vi "Actor Core.vi"(8 "error in":errorcluster, 11 "Algorythm in":refnum<class "Algorythm.lvclass">) -> (0 "error out":errorcluster, 3 "Actor out":refnum<class "Actor.lvclass">)   [LabVIEW 2020, in "Algorythm.lvlib" / "Algorythm.lvclass"]
doc: "(<B>Filename</B>: Actor Framework.lvlib:Actor.lvclass:Actor Core.vi)\n\nReceives messages to the actor, reacts to them, and initiates any error handling that may shut the actor down.\n\nDescendant classes may override this VI to append parallel tasks for the actor to complete while it handles messages. Overrides use the Call Parent Class Method node."
uses:
  Algorythm.lvclass
  C:/Program Files (x86)/National Instruments/LabVIEW 2020/vi.lib/ActorFramework/Actor/Actor.lvclass
  <vilib>/ActorFramework/Actor/Actor.lvclass
  <vilib>/ActorFramework/Actor/Actor.lvclass/Actor.ctl
  <vilib>/ActorFramework/Message Enqueuer/Message Enqueuer.lvclass/Message Enqueuer.ctl
  Algorythm.lvclass/Algorythm.ctl
  <vilib>/Platform/TimedLoop/XDataNode/timing_clust.ctl
  <vilib>/Platform/TimedLoop/XDataNode/nitl_modes.ctl
  <vilib>/Platform/TimedLoop/XDataNode/wakeup.ctl
  Modbus/Modbus Messages/Write to Module Msg/Write to Module Msg.lvclass/Write to Module Msg.ctl
  GUI Messages/Get Alg Result Msg/Get Alg Result Msg.lvclass/Get Alg Result Msg.ctl
  <vilib>/ActorFramework/Message Enqueuer/Init from Existing Queue.vi
  <vilib>/ActorFramework/Message Enqueuer/Enqueue.vi
  Modbus/Modbus Messages/Write to Module Msg/Write to Module Msg.lvclass
  C:/Program Files (x86)/National Instruments/LabVIEW 2020/vi.lib/ActorFramework/Message/Message.lvclass
  GUI Messages/Get Alg Result Msg/Get Alg Result Msg.lvclass
  <vilib>/ActorFramework/Stop Msg/Stop Msg.lvclass
  <vilib>/Platform/TimedLoop/scheduler/LVUserAPI/_suppVIs/Create_1kHz_TSource.vi
  <vilib>/Utility/LVClass/Get LV Class Name.vi
  <resource>/AFDebug/Generate Trace for Message.vi
  <vilib>/ActorFramework/Message Priority Queue/Priority Enqueue.vi
  <vilib>/ActorFramework/Message Enqueuer/Message Enqueuer.lvclass
  <vilib>/platform/TimedLoop/XDataNode/XDataNode.xnode
  <vilib>/Platform/TimedLoop/XDataNode/XDNodeRunTimeDep.lvlib
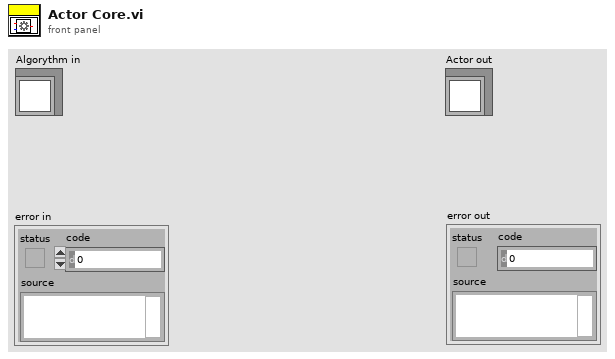
[diagram p1: front panel]
types:
  T1 = cluster{"Relay 1":bool, "Relay 2":bool, "Relay 3":bool, "Relay 4":bool, "Relay 5":bool, "Relay 6":bool, "Relay 7":bool, "Relay 8":bool}
  T2 = typedef "XDNodeRunTimeDep.lvlib/timing_clust.ctl" = cluster{"Expected End [f-1]":u64, "Actual End [f-1]":u64, "Finished Late? [f-1]":bool, "Expected End [i-1]":u64, "Actual End [i-1]":u64, "Finished Late? [i-1]":bool, "Expected Start [i]":u64, "Actual Start [i]":u64, "Expected Start [f]":u64, "Actual Start [f]":u64, "Source Name":string, "Structure Name":string, "Period":i64, "Deadline":i64, "Offset":i64, "Start":i64, "Priority":i32, "Timeout":i32, "Mode":T3, "Wakeup Reason":T4, "Error":errorcluster, "Source Type":string, "Secondary Source Type":string, "Global End Time":u64, "Global Start Time":u64, "Frame Duration":u64, "Iteration Duration":u64, "Assigned CPU":i32, "I/O Scan Engine Mode":u32}
  T3 = typedef "XDNodeRunTimeDep.lvlib/nitl_modes.ctl" = enum32{"No Change", "Process missed periods, maintain original phase", "Discard missed periods, maintain original phase", "Process missed periods, ignore original phase", "Discard missed periods, ignore original phase"}
  T4 = typedef "XDNodeRunTimeDep.lvlib/wakeup.ctl" = enum32{"Normal", "Aborted", "Asynchronous wakeup", "Timing source error", "Timed loop error", "Timeout"}
  T5 = cluster{"LDO":i32, "LAI":i32, "Control":i32, "Connect":i32}
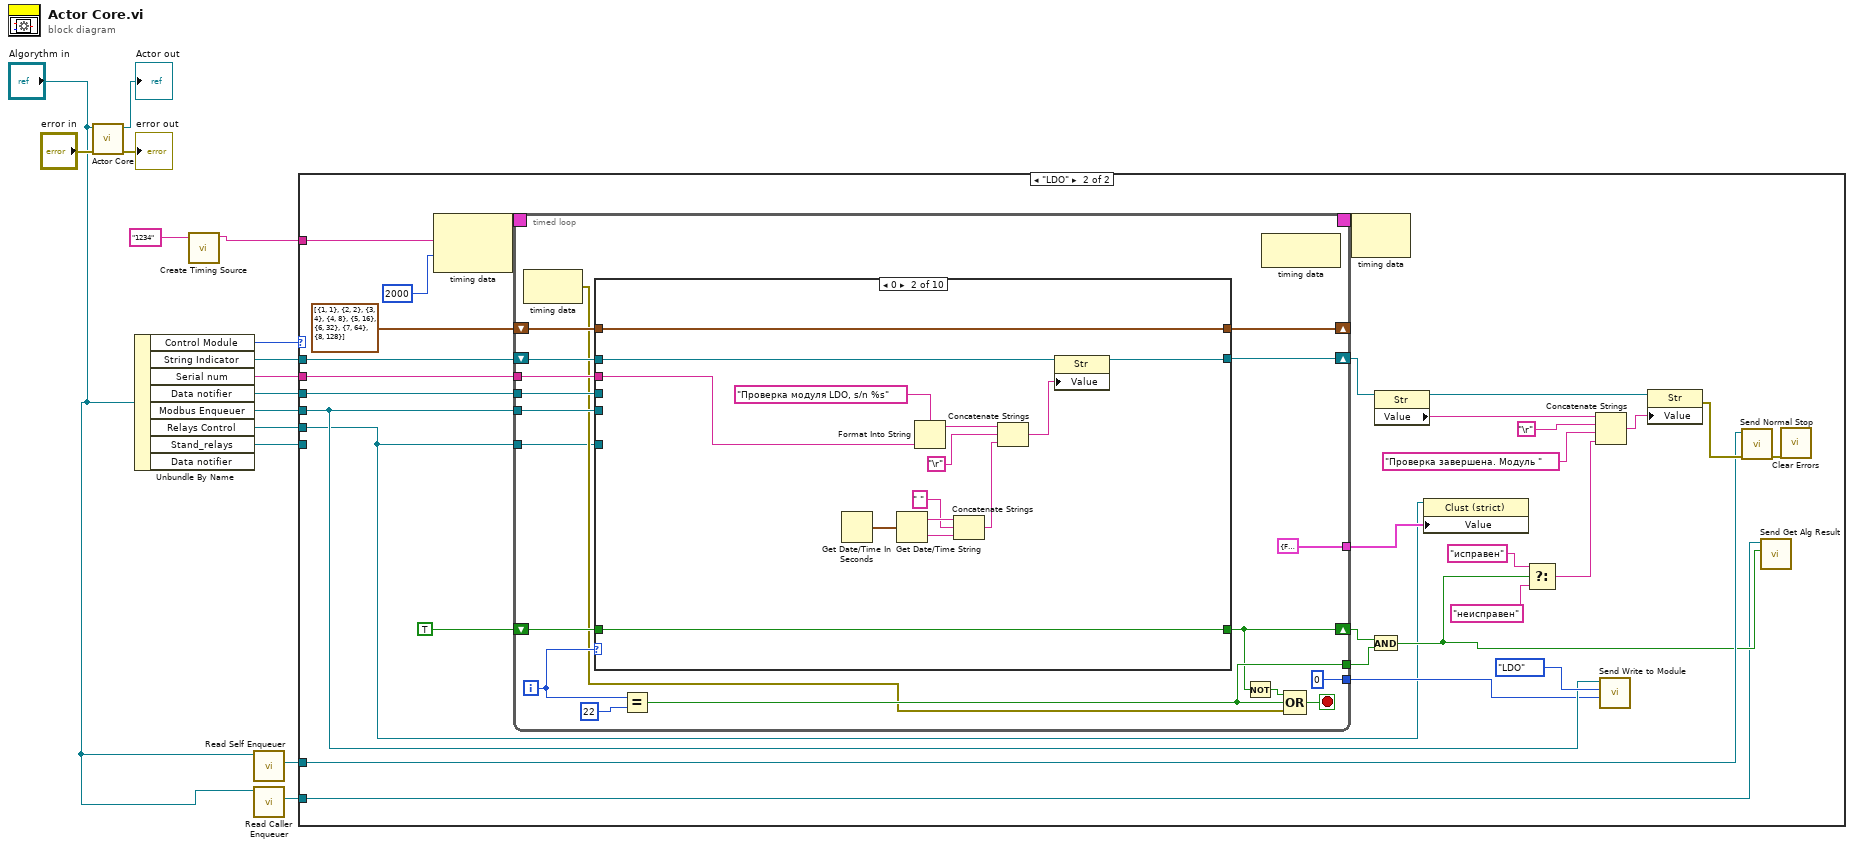
[diagram p0: block diagram]
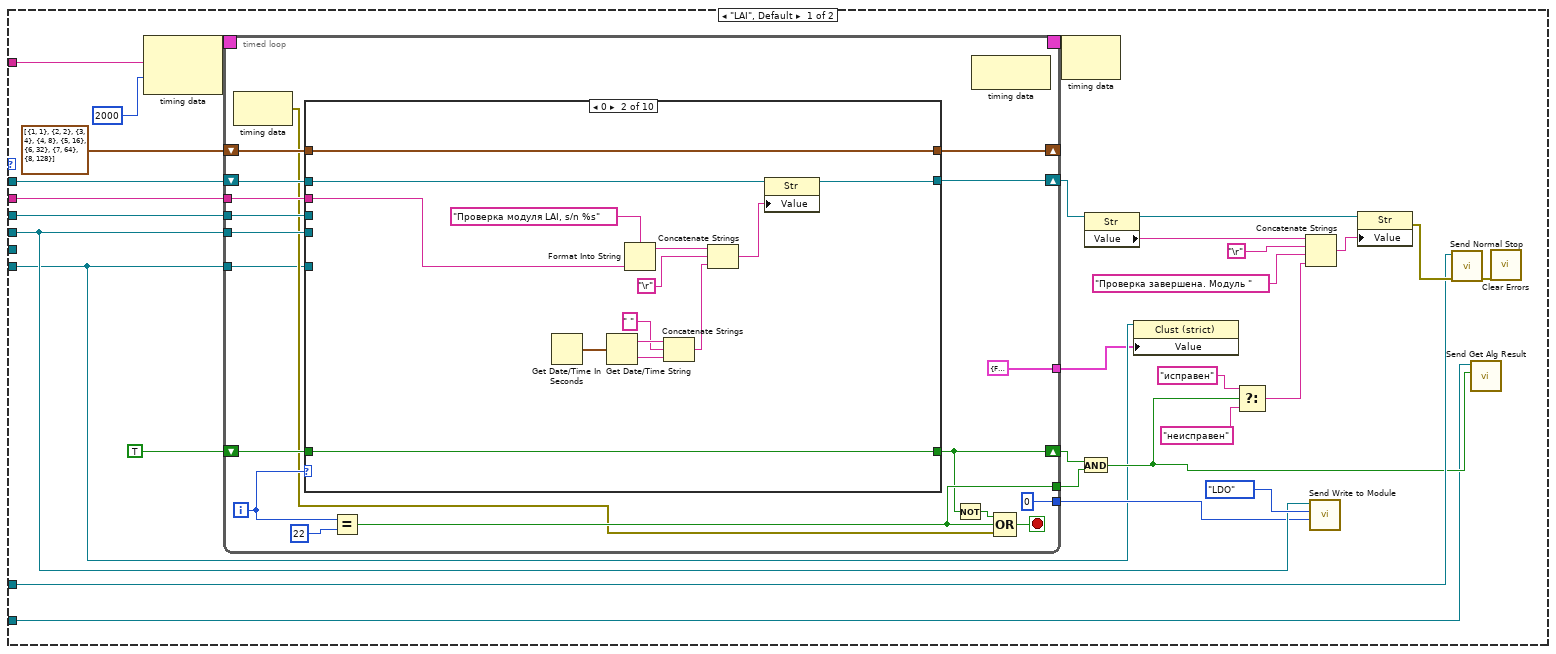
[diagram p2: hidden frame]
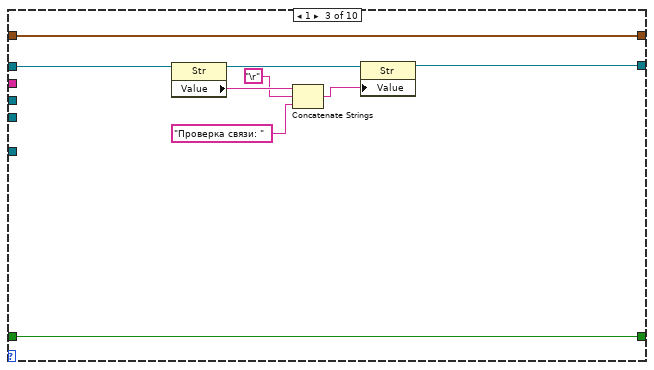
[diagram p4: hidden frame]
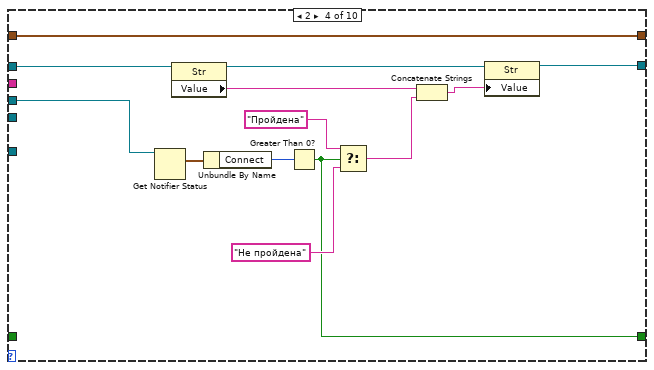
[diagram p5: hidden frame]
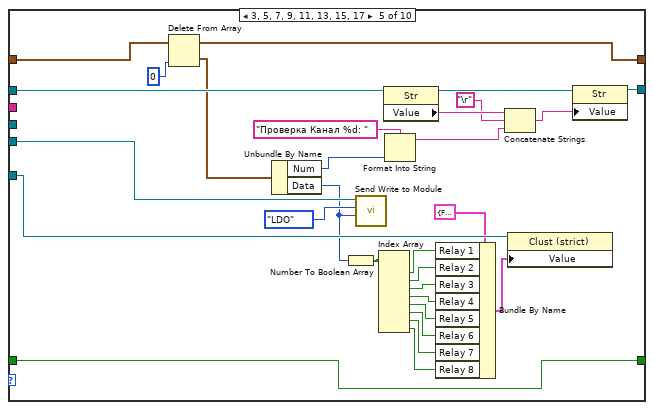
[diagram p6: hidden frame]
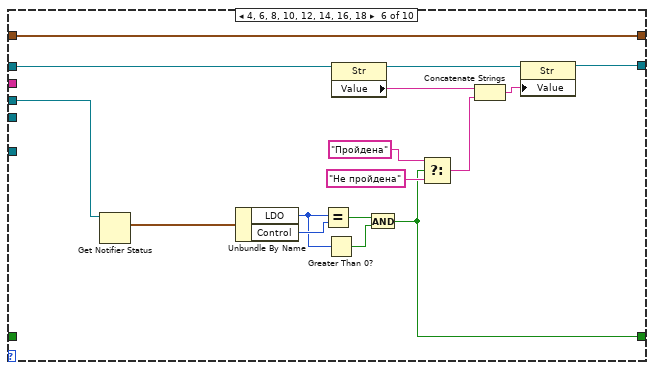
[diagram p7: hidden frame]
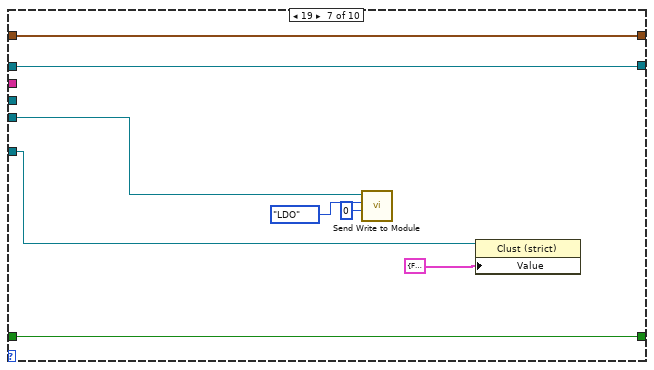
[diagram p8: hidden frame]
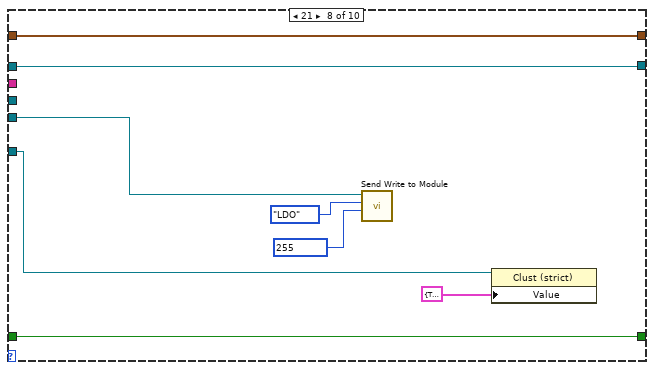
[diagram p9: hidden frame]
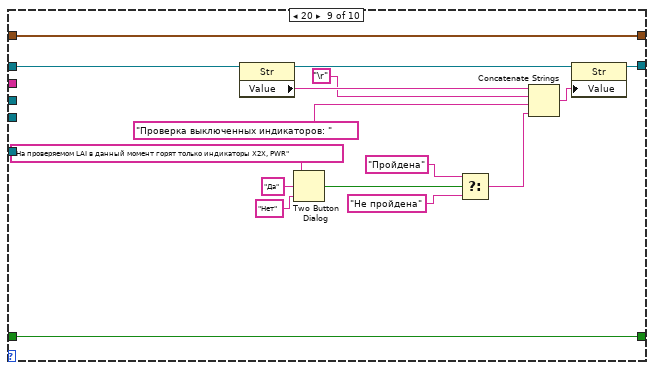
[diagram p10: hidden frame]
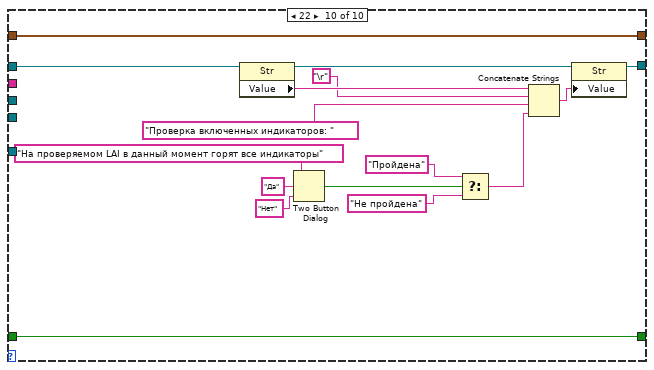
[diagram p11: hidden frame]
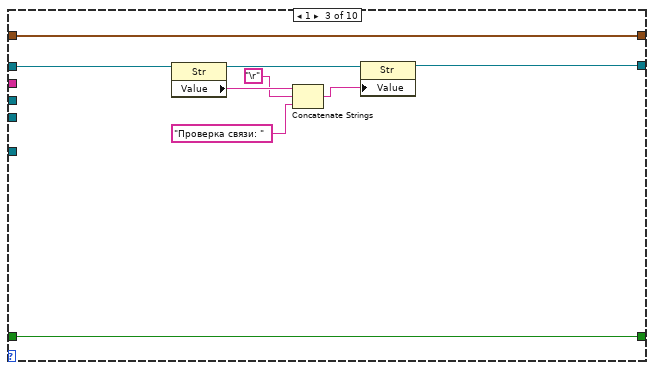
[diagram p13: hidden frame]
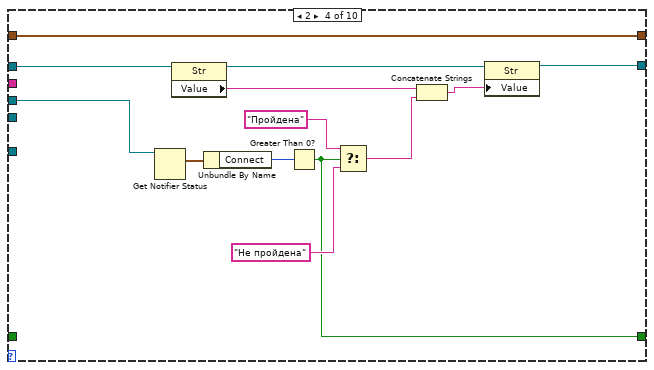
[diagram p14: hidden frame]
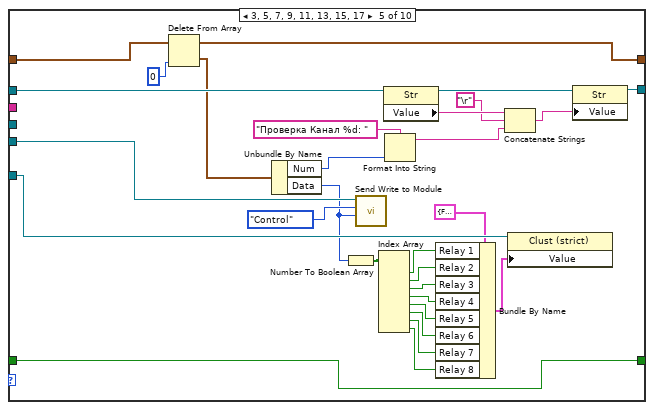
[diagram p15: hidden frame]
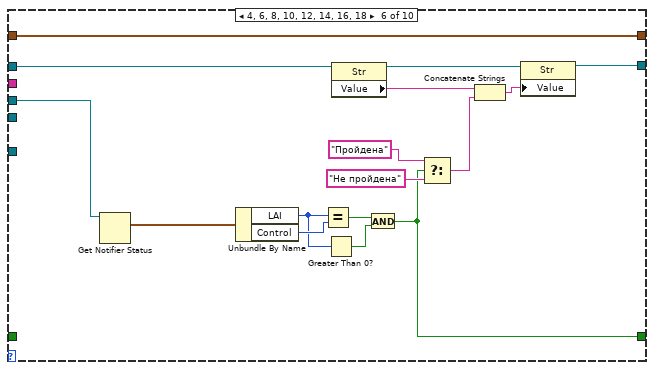
[diagram p16: hidden frame]
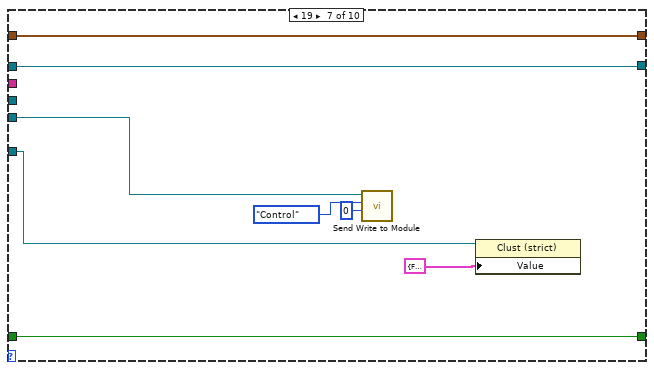
[diagram p17: hidden frame]
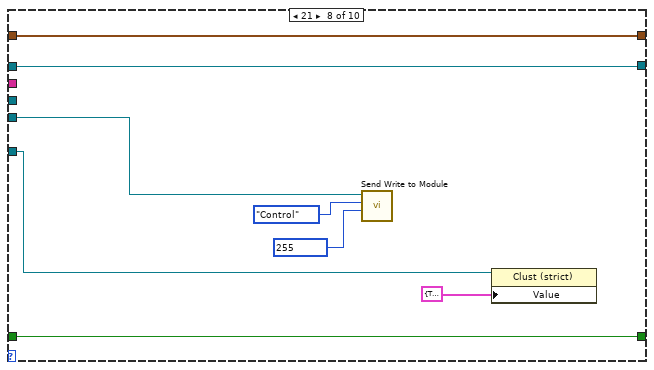
[diagram p18: hidden frame]
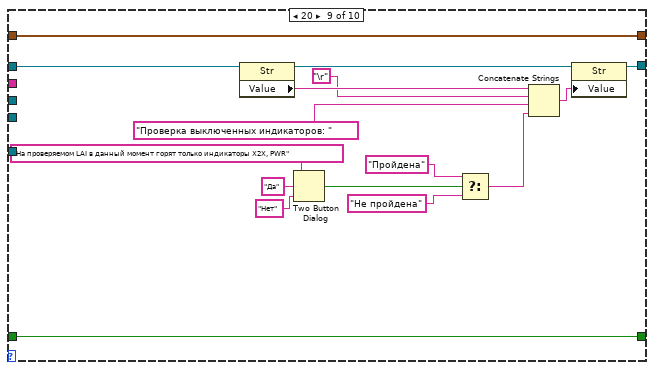
[diagram p19: hidden frame]
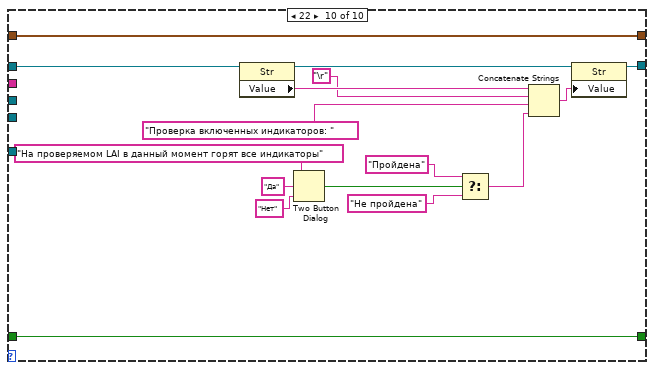
[diagram p20: hidden frame]
diagram:
  n1 = call-parent "Actor Core.vi"("error in"="error in", "Actor in"="Algorythm in") -> ("error out"=→"error out":errorcluster, "Actor out"=→"Actor out":refnum<class "Actor.lvclass">)  [unwired: 8 in]
  n2 = Unbundle By Name("Algorythm in") -> ("Control Module"=w12:enum16{"LAI", "LDO"}, "String Indicator"=w11:refnum<vi>, "Serial num"=w10:string, "Data notifier"=w9:refnum<notifier>, "Modbus Enqueuer"=w8:refnum<class "Message Enqueuer.lvclass">, "Relays Control"=w1:refnum<vi>, "Stand_relays"=w2:refnum<vi>)  [unwired: 1 out]
  n3 = call-poly <vilib>:"Create Timing Source.vi"("name (in)"="1234") -> ("name (out)"=w5:string)  [unwired: 9 in, 1 out]
  n4 = call <vilib>:"Read Self Enqueuer.vi"("Actor"="Algorythm in") -> ("Self Enqueuer"=w7:refnum<class "Message Enqueuer.lvclass">)  [unwired: 10 in]
  n5 = call <vilib>:"Read Caller Enqueuer.vi"("Actor"="Algorythm in") -> ("Caller Enqueuer"=w3:refnum<class "Message Enqueuer.lvclass">)  [unwired: 10 in]
  n6 = case shown="\"LDO\"" w12 {
    tunnel: w11 -> [w34 w222]
    tunnel: w10 -> [w42 w230]
    tunnel: w9 -> [w41 w229]
    tunnel: w8 -> [w19 w207]
    tunnel: w7 -> [w25 w213]
    tunnel: w5 -> [w23 w211]
    tunnel: w3 -> [w21 w209]
    tunnel: w2 -> [w17 _]
    tunnel: w1 -> [_ w204]
    frame "LAI", Default {
      n7 = node-c288(w23, i64 2000 ("Period")) -> (w45:T2)
      n8 = timed-loop {
        timing: w45 -> [_]
        timing-out: [_] -> w44
        tunnel: w42 -> [w62]
        tunnel: w41 -> [w61]
        shift-right: [w46] -> w33
        shift-left: TRUE -> [w60]
        tunnel: w19 -> [w59]
        shift-right: [w58] -> _
        shift-left: cluster{"Num":u16, "Data":u16}[] [{"Num"=1, "Data"=1}, {"Num"=2, "Data"=2}, {"Num"=3, "Data"=4}, {"Num"=4, "Data"=8}, {"Num"=5, "Data"=16}, {"Num"=6, "Data"=32}, {"Num"=7, "Data"=64}, {"Num"=8, "Data"=128}] -> [w57]
        tunnel: [w53] -> w32
        shift-right: [w52] -> w27
        shift-left: w34 -> [w63]
        tunnel: [u16 0 ("Data")] -> w18
        tunnel: w17 -> [w49]
        tunnel: [T1 {"Relay 1"=FALSE, "Relay 2"=FALSE, "Relay 3"=FALSE, "Relay 4"=FALSE, "Relay 5"=FALSE, "Relay 6"=FALSE, "Relay 7"=FALSE, "Relay 8"=FALSE} ("Value")] -> w16
        i -> [w56]
        stop <- w54 stop-if-true
        n9 = node-c288() -> (w51:errorcluster)  [unwired: 1 in]
        n10 = case shown="0" w56 {
          tunnel: w63 -> [w64 w80 w89 w102 w128 w143 w150 w158 w173 w189]
          tunnel: w62 -> [_ w78 _ _ _ _ _ _ _ _]
          tunnel: w61 -> [_ _ _ w92 _ w133 _ _ _ _]
          tunnel: [w66 w77 w83 w95 w113 w137 w155 w163 w179 w195] -> w46
          tunnel: w60 -> [w66 w77 w83 _ w113 _ w155 w163 w179 w195]
          tunnel: w59 -> [_ _ _ _ w126 _ w152 w160 _ _]
          tunnel: [w65 w76 w82 w94 w123 w147 w154 w162 w178 w194] -> w58
          tunnel: w57 -> [w65 w76 w82 w94 w124 w147 w154 w162 w178 w194]
          tunnel: [w64 w75 w81 w93 w117 w136 w150 w158 w164 w180] -> w52
          tunnel: w49 -> [_ _ _ _ w116 _ w149 w156 _ _]
          frame -1, Default {
          }
          frame 0 {
            n11 = Get Date/Time In Seconds() -> (seconds since 1Jan1904=w72:timestamp)
            n12 = Get Date/Time String(seconds (now)=w72) -> (date string=w71:string, time string=w69:string)  [unwired: 2 in]
            n13 = Format Into String(format string="Проверка модуля LAI, s/n %s", w78) -> (resulting string=w74:string)  [unwired: 2 in, 1 out]
            n14 = Concatenate Strings(w71, " " ("string"), w69) -> (w68:string)
            n15 = Concatenate Strings(w74, "\r", w68) -> (w67:string)
            n16 = property class="Str"(reference=w80, "Value"=w67) -> (reference out=w75:refnum<vi>)  [unwired: 1 in, 1 out]
          }
          frame 1 {
            n17 = property class="Str"(reference=w89) -> (reference out=w88:refnum<vi>, "Value"=w87:string)  [unwired: 1 in, 1 out]
            n18 = Concatenate Strings(w87, "\r", "Проверка связи: " ("string")) -> (w85:string)
            n19 = property class="Str"(reference=w88, "Value"=w85) -> (reference out=w81:refnum<vi>)  [unwired: 1 in, 1 out]
          }
          frame 2 {
            n20 = Get Notifier Status(notifier=w92) -> (current notification=w91:T5)  [unwired: 1 in, 4 out]
            n21 = property class="Str"(reference=w102) -> (reference out=w101:refnum<vi>, "Value"=w100:string)  [unwired: 1 in, 1 out]
            n22 = Unbundle By Name(w91) -> ("Connect"=w90:i32)
            n23 = Greater Than 0?(x=w90) -> (x > 0?=w95:bool)
            n24 = Select(t="Пройдена" ("string"), s=w95, f="Не пройдена" ("string")) -> (s? t:f=w96:string)
            n25 = Concatenate Strings(w100, w96) -> (w99:string)
            n26 = property class="Str"(reference=w101, "Value"=w99) -> (reference out=w93:refnum<vi>)  [unwired: 1 in, 1 out]
          }
          frame 3, 5, 7, 9, 11, 13, 15, 17 {
            n27 = Delete From Array(array=w124, index=0) -> (deleted portion=w118:cluster{"Num":u16, "Data":u16}, array with subset deleted=w123:cluster{"Num":u16, "Data":u16}[])  [unwired: 1 in]
            n28 = Unbundle By Name(w118) -> ("Num"=w119:u16, "Data"=w115:u16)
            n29 = Number To Boolean Array(number=w115) -> (Boolean array=w112:bool[])
            n30 = call "Send Write to Module.vi"("Data"=w115, "Module"=enum16{"LAI", "LDO", "Control"}."LDO", "Message Enqueuer"=w126) -> ()  [unwired: 7 in, 2 out]
            n31 = Index Array(array=w112) -> (element #1=w111:bool, element #2=w110:bool, element #3=w109:bool, element #4=w108:bool, element #5=w107:bool, element #6=w106:bool, element #7=w105:bool, element #8=w104:bool)  [unwired: 8 in]
            n32 = property class="Str"(reference=w128) -> (reference out=w131:refnum<vi>, "Value"=w130:string)  [unwired: 1 in, 1 out]
            n33 = Format Into String(format string="Проверка Канал %d: ", w119) -> (resulting string=w120:string)  [unwired: 2 in, 1 out]
            n34 = Bundle By Name(cluster=T1 {"Relay 1"=FALSE, "Relay 2"=FALSE, "Relay 3"=FALSE, "Relay 4"=FALSE, "Relay 5"=FALSE, "Relay 6"=FALSE, "Relay 7"=FALSE, "Relay 8"=FALSE} ("Value"), "Relay 1"=w111, "Relay 2"=w110, "Relay 3"=w109, "Relay 4"=w108, "Relay 5"=w107, "Relay 6"=w106, "Relay 7"=w105, "Relay 8"=w104) -> (w103:T1)
            n35 = Concatenate Strings(w130, "\r", w120) -> (w129:string)
            n36 = property class="Clust (strict)"(reference=w116, "Value"=w103) -> ()  [unwired: 1 in, 2 out]
            n37 = property class="Str"(reference=w131, "Value"=w129) -> (reference out=w117:refnum<vi>)  [unwired: 1 in, 1 out]
          }
          frame 4, 6, 8, 10, 12, 14, 16, 18 {
            n38 = Get Notifier Status(notifier=w133) -> (current notification=w132:T5)  [unwired: 1 in, 4 out]
            n39 = Unbundle By Name(w132) -> ("LDO"=w134:i32, "Control"=w135:i32)
            n40 = Equal?(x=w134, y=w135) -> (x = y?=w139:bool)
            n41 = Greater Than 0?(x=w134) -> (x > 0?=w138:bool)
            n42 = property class="Str"(reference=w143) -> (reference out=w146:refnum<vi>, "Value"=w145:string)  [unwired: 1 in, 1 out]
            n43 = And(x=w139, y=w138) -> (x .and. y?=w137:bool)
            n44 = Select(t="Пройдена" ("string"), s=w137, f="Не пройдена" ("string")) -> (s? t:f=w140:string)
            n45 = Concatenate Strings(w145, w140) -> (w144:string)
            n46 = property class="Str"(reference=w146, "Value"=w144) -> (reference out=w136:refnum<vi>)  [unwired: 1 in, 1 out]
          }
          frame 19 {
            n47 = call "Send Write to Module.vi"("Data"=u16 0, "Module"=enum16{"LAI", "LDO", "Control"}."LDO", "Message Enqueuer"=w152) -> ()  [unwired: 7 in, 2 out]
            n48 = property class="Clust (strict)"(reference=w149, "Value"=T1 {"Relay 1"=FALSE, "Relay 2"=FALSE, "Relay 3"=FALSE, "Relay 4"=FALSE, "Relay 5"=FALSE, "Relay 6"=FALSE, "Relay 7"=FALSE, "Relay 8"=FALSE}) -> ()  [unwired: 1 in, 2 out]
          }
          frame 21 {
            n49 = call "Send Write to Module.vi"("Data"=u16 255, "Module"=enum16{"LAI", "LDO", "Control"}."LDO", "Message Enqueuer"=w160) -> ()  [unwired: 7 in, 2 out]
            n50 = property class="Clust (strict)"(reference=w156, "Value"=T1 {"Relay 1"=TRUE, "Relay 2"=TRUE, "Relay 3"=TRUE, "Relay 4"=TRUE, "Relay 5"=TRUE, "Relay 6"=TRUE, "Relay 7"=TRUE, "Relay 8"=TRUE}) -> ()  [unwired: 1 in, 2 out]
          }
          frame 20 {
            n51 = property class="Str"(reference=w173) -> (reference out=w177:refnum<vi>, "Value"=w176:string)  [unwired: 1 in, 1 out]
            n52 = Two Button Dialog(message="На проверяемом LAI в данный момент горят только индикаторы X2X, PWR", 1:"Нет" ("T button name (\"OK\")"), 2:"Да" ("T button name (\"OK\")")) -> (T button?=w168:bool)
            n53 = Select(t="Пройдена" ("T button name (\"OK\")"), s=w168, f="Не пройдена" ("T button name (\"OK\")")) -> (s? t:f=w165:string)
            n54 = Concatenate Strings(w176, "\r", "Проверка выключенных индикаторов: " ("string"), w165) -> (w175:string)
            n55 = property class="Str"(reference=w177, "Value"=w175) -> (reference out=w164:refnum<vi>)  [unwired: 1 in, 1 out]
          }
          frame 22 {
            n56 = property class="Str"(reference=w189) -> (reference out=w193:refnum<vi>, "Value"=w192:string)  [unwired: 1 in, 1 out]
            n57 = Two Button Dialog(message="На проверяемом LAI в данный момент горят все индикаторы", 1:"Нет" ("T button name (\"OK\")"), 2:"Да" ("T button name (\"OK\")")) -> (T button?=w184:bool)
            n58 = Select(t="Пройдена" ("T button name (\"OK\")"), s=w184, f="Не пройдена" ("T button name (\"OK\")")) -> (s? t:f=w181:string)
            n59 = Concatenate Strings(w192, "\r", "Проверка включенных индикаторов: " ("string"), w181) -> (w191:string)
            n60 = property class="Str"(reference=w193, "Value"=w191) -> (reference out=w180:refnum<vi>)  [unwired: 1 in, 1 out]
          }
        }
        n61 = Equal?(x=w56, y=22) -> (x = y?=w53:bool)
        n62 = Not(x=w46) -> (.not. x?=w47:bool)
        n63 = node-c288() -> ()  [unwired: 1 in, 1 out]
        n64 = Compound Arithmetic op=OR(w47, w53, w51) -> (w54:bool)
      }
      n65 = node-c288(w44) -> ()  [unwired: 1 out]
      n66 = And(x=w33, y=w32) -> (x .and. y?=w22:bool)
      n67 = property class="Str"(reference=w27) -> (reference out=w28:refnum<vi>, "Value"=w38:string)  [unwired: 1 in, 1 out]
      n68 = property class="Clust (strict)"(reference=w17, "Value"=w16) -> ()  [unwired: 1 in, 2 out]
      n69 = Select(t="исправен" ("string"), s=w22, f="неисправен" ("string")) -> (s? t:f=w29:string)
      n70 = Concatenate Strings(w38, "\r", "Проверка завершена. Модуль " ("string"), w29) -> (w37:string)
      n71 = call "Send Write to Module.vi"("Data"=w18, "Module"=enum16{"LAI", "LDO", "Control"}."LDO", "Message Enqueuer"=w19) -> ()  [unwired: 7 in, 2 out]
      n72 = property class="Str"(reference=w28, "Value"=w37) -> (error out=w26:errorcluster)  [unwired: 1 in, 1 out]
      n73 = call <vilib>:"Send Normal Stop.vi"("error in (no error)"=w26, "Message Enqueuer"=w25) -> ("error out"=w24:errorcluster)  [unwired: 9 in]
      n74 = call "Send Get Alg Result.vi"("Alg result"=w22, "Message Enqueuer"=w21) -> ()  [unwired: 8 in, 2 out]
      n75 = call <vilib>:"Clear Errors.vi"("error in (no error)"=w24) -> ()  [unwired: 5 in, 2 out]
    }
    frame "LDO" {
      n76 = node-c288(w211, i64 2000 ("Period")) -> (w233:T2)
      n77 = timed-loop {
        timing: w233 -> [_]
        timing-out: [_] -> w232
        tunnel: w230 -> [w250]
        tunnel: w229 -> [w249]
        shift-right: [w234] -> w221
        shift-left: TRUE -> [w248]
        tunnel: w207 -> [w247]
        shift-right: [w246] -> _
        shift-left: cluster{"Num":u16, "Data":u16}[] [{"Num"=1, "Data"=1}, {"Num"=2, "Data"=2}, {"Num"=3, "Data"=4}, {"Num"=4, "Data"=8}, {"Num"=5, "Data"=16}, {"Num"=6, "Data"=32}, {"Num"=7, "Data"=64}, {"Num"=8, "Data"=128}] -> [w245]
        tunnel: [w241] -> w220
        shift-right: [w240] -> w215
        shift-left: w222 -> [w251]
        tunnel: [u16 0 ("Data")] -> w206
        tunnel: w204 -> [w237]
        tunnel: [T1 {"Relay 1"=FALSE, "Relay 2"=FALSE, "Relay 3"=FALSE, "Relay 4"=FALSE, "Relay 5"=FALSE, "Relay 6"=FALSE, "Relay 7"=FALSE, "Relay 8"=FALSE} ("Value")] -> w205
        i -> [w244]
        stop <- w242 stop-if-true
        n78 = node-c288() -> (w239:errorcluster)  [unwired: 1 in]
        n79 = case shown="0" w244 {
          tunnel: w251 -> [w252 w268 w277 w290 w316 w331 w338 w346 w361 w377]
          tunnel: w250 -> [_ w266 _ _ _ _ _ _ _ _]
          tunnel: w249 -> [_ _ _ w280 _ w321 _ _ _ _]
          tunnel: [w254 w265 w271 w283 w301 w325 w343 w351 w367 w383] -> w234
          tunnel: w248 -> [w254 w265 w271 _ w301 _ w343 w351 w367 w383]
          tunnel: w247 -> [_ _ _ _ w314 _ w340 w348 _ _]
          tunnel: [w253 w264 w270 w282 w311 w335 w342 w350 w366 w382] -> w246
          tunnel: w245 -> [w253 w264 w270 w282 w312 w335 w342 w350 w366 w382]
          tunnel: [w252 w263 w269 w281 w305 w324 w338 w346 w352 w368] -> w240
          tunnel: w237 -> [_ _ _ _ w304 _ w337 w344 _ _]
          frame -1, Default {
          }
          frame 0 {
            n80 = Get Date/Time In Seconds() -> (seconds since 1Jan1904=w260:timestamp)
            n81 = Get Date/Time String(seconds (now)=w260) -> (date string=w259:string, time string=w257:string)  [unwired: 2 in]
            n82 = Format Into String(format string="Проверка модуля LDO, s/n %s", w266) -> (resulting string=w262:string)  [unwired: 2 in, 1 out]
            n83 = Concatenate Strings(w259, " " ("string"), w257) -> (w256:string)
            n84 = Concatenate Strings(w262, "\r", w256) -> (w255:string)
            n85 = property class="Str"(reference=w268, "Value"=w255) -> (reference out=w263:refnum<vi>)  [unwired: 1 in, 1 out]
          }
          frame 1 {
            n86 = property class="Str"(reference=w277) -> (reference out=w276:refnum<vi>, "Value"=w275:string)  [unwired: 1 in, 1 out]
            n87 = Concatenate Strings(w275, "\r", "Проверка связи: " ("string")) -> (w273:string)
            n88 = property class="Str"(reference=w276, "Value"=w273) -> (reference out=w269:refnum<vi>)  [unwired: 1 in, 1 out]
          }
          frame 2 {
            n89 = Get Notifier Status(notifier=w280) -> (current notification=w279:T5)  [unwired: 1 in, 4 out]
            n90 = property class="Str"(reference=w290) -> (reference out=w289:refnum<vi>, "Value"=w288:string)  [unwired: 1 in, 1 out]
            n91 = Unbundle By Name(w279) -> ("Connect"=w278:i32)
            n92 = Greater Than 0?(x=w278) -> (x > 0?=w283:bool)
            n93 = Select(t="Пройдена" ("string"), s=w283, f="Не пройдена" ("string")) -> (s? t:f=w284:string)
            n94 = Concatenate Strings(w288, w284) -> (w287:string)
            n95 = property class="Str"(reference=w289, "Value"=w287) -> (reference out=w281:refnum<vi>)  [unwired: 1 in, 1 out]
          }
          frame 3, 5, 7, 9, 11, 13, 15, 17 {
            n96 = Delete From Array(array=w312, index=0) -> (deleted portion=w306:cluster{"Num":u16, "Data":u16}, array with subset deleted=w311:cluster{"Num":u16, "Data":u16}[])  [unwired: 1 in]
            n97 = Unbundle By Name(w306) -> ("Num"=w307:u16, "Data"=w303:u16)
            n98 = Number To Boolean Array(number=w303) -> (Boolean array=w300:bool[])
            n99 = call "Send Write to Module.vi"("Data"=w303, "Module"=enum16{"LAI", "LDO", "Control"}."Control", "Message Enqueuer"=w314) -> ()  [unwired: 7 in, 2 out]
            n100 = Index Array(array=w300) -> (element #1=w299:bool, element #2=w298:bool, element #3=w297:bool, element #4=w296:bool, element #5=w295:bool, element #6=w294:bool, element #7=w293:bool, element #8=w292:bool)  [unwired: 8 in]
            n101 = property class="Str"(reference=w316) -> (reference out=w319:refnum<vi>, "Value"=w318:string)  [unwired: 1 in, 1 out]
            n102 = Format Into String(format string="Проверка Канал %d: ", w307) -> (resulting string=w308:string)  [unwired: 2 in, 1 out]
            n103 = Bundle By Name(cluster=T1 {"Relay 1"=FALSE, "Relay 2"=FALSE, "Relay 3"=FALSE, "Relay 4"=FALSE, "Relay 5"=FALSE, "Relay 6"=FALSE, "Relay 7"=FALSE, "Relay 8"=FALSE} ("Value"), "Relay 1"=w299, "Relay 2"=w298, "Relay 3"=w297, "Relay 4"=w296, "Relay 5"=w295, "Relay 6"=w294, "Relay 7"=w293, "Relay 8"=w292) -> (w291:T1)
            n104 = Concatenate Strings(w318, "\r", w308) -> (w317:string)
            n105 = property class="Clust (strict)"(reference=w304, "Value"=w291) -> ()  [unwired: 1 in, 2 out]
            n106 = property class="Str"(reference=w319, "Value"=w317) -> (reference out=w305:refnum<vi>)  [unwired: 1 in, 1 out]
          }
          frame 4, 6, 8, 10, 12, 14, 16, 18 {
            n107 = Get Notifier Status(notifier=w321) -> (current notification=w320:T5)  [unwired: 1 in, 4 out]
            n108 = Unbundle By Name(w320) -> ("LAI"=w322:i32, "Control"=w323:i32)
            n109 = Equal?(x=w322, y=w323) -> (x = y?=w327:bool)
            n110 = Greater Than 0?(x=w322) -> (x > 0?=w326:bool)
            n111 = property class="Str"(reference=w331) -> (reference out=w334:refnum<vi>, "Value"=w333:string)  [unwired: 1 in, 1 out]
            n112 = And(x=w327, y=w326) -> (x .and. y?=w325:bool)
            n113 = Select(t="Пройдена" ("string"), s=w325, f="Не пройдена" ("string")) -> (s? t:f=w328:string)
            n114 = Concatenate Strings(w333, w328) -> (w332:string)
            n115 = property class="Str"(reference=w334, "Value"=w332) -> (reference out=w324:refnum<vi>)  [unwired: 1 in, 1 out]
          }
          frame 19 {
            n116 = call "Send Write to Module.vi"("Data"=u16 0, "Module"=enum16{"LAI", "LDO", "Control"}."Control", "Message Enqueuer"=w340) -> ()  [unwired: 7 in, 2 out]
            n117 = property class="Clust (strict)"(reference=w337, "Value"=T1 {"Relay 1"=FALSE, "Relay 2"=FALSE, "Relay 3"=FALSE, "Relay 4"=FALSE, "Relay 5"=FALSE, "Relay 6"=FALSE, "Relay 7"=FALSE, "Relay 8"=FALSE}) -> ()  [unwired: 1 in, 2 out]
          }
          frame 21 {
            n118 = call "Send Write to Module.vi"("Data"=u16 255, "Module"=enum16{"LAI", "LDO", "Control"}."Control", "Message Enqueuer"=w348) -> ()  [unwired: 7 in, 2 out]
            n119 = property class="Clust (strict)"(reference=w344, "Value"=T1 {"Relay 1"=TRUE, "Relay 2"=TRUE, "Relay 3"=TRUE, "Relay 4"=TRUE, "Relay 5"=TRUE, "Relay 6"=TRUE, "Relay 7"=TRUE, "Relay 8"=TRUE}) -> ()  [unwired: 1 in, 2 out]
          }
          frame 20 {
            n120 = property class="Str"(reference=w361) -> (reference out=w365:refnum<vi>, "Value"=w364:string)  [unwired: 1 in, 1 out]
            n121 = Two Button Dialog(message="На проверяемом LAI в данный момент горят только индикаторы X2X, PWR", 1:"Нет" ("T button name (\"OK\")"), 2:"Да" ("T button name (\"OK\")")) -> (T button?=w356:bool)
            n122 = Select(t="Пройдена" ("T button name (\"OK\")"), s=w356, f="Не пройдена" ("T button name (\"OK\")")) -> (s? t:f=w353:string)
            n123 = Concatenate Strings(w364, "\r", "Проверка выключенных индикаторов: " ("string"), w353) -> (w363:string)
            n124 = property class="Str"(reference=w365, "Value"=w363) -> (reference out=w352:refnum<vi>)  [unwired: 1 in, 1 out]
          }
          frame 22 {
            n125 = property class="Str"(reference=w377) -> (reference out=w381:refnum<vi>, "Value"=w380:string)  [unwired: 1 in, 1 out]
            n126 = Two Button Dialog(message="На проверяемом LAI в данный момент горят все индикаторы", 1:"Нет" ("T button name (\"OK\")"), 2:"Да" ("T button name (\"OK\")")) -> (T button?=w372:bool)
            n127 = Select(t="Пройдена" ("T button name (\"OK\")"), s=w372, f="Не пройдена" ("T button name (\"OK\")")) -> (s? t:f=w369:string)
            n128 = Concatenate Strings(w380, "\r", "Проверка включенных индикаторов: " ("string"), w369) -> (w379:string)
            n129 = property class="Str"(reference=w381, "Value"=w379) -> (reference out=w368:refnum<vi>)  [unwired: 1 in, 1 out]
          }
        }
        n130 = Equal?(x=w244, y=22) -> (x = y?=w241:bool)
        n131 = Not(x=w234) -> (.not. x?=w235:bool)
        n132 = node-c288() -> ()  [unwired: 1 in, 1 out]
        n133 = Compound Arithmetic op=OR(w235, w241, w239) -> (w242:bool)
      }
      n134 = node-c288(w232) -> ()  [unwired: 1 out]
      n135 = And(x=w221, y=w220) -> (x .and. y?=w210:bool)
      n136 = property class="Str"(reference=w215) -> (reference out=w216:refnum<vi>, "Value"=w226:string)  [unwired: 1 in, 1 out]
      n137 = property class="Clust (strict)"(reference=w204, "Value"=w205) -> ()  [unwired: 1 in, 2 out]
      n138 = Select(t="исправен" ("string"), s=w210, f="неисправен" ("string")) -> (s? t:f=w217:string)
      n139 = Concatenate Strings(w226, "\r", "Проверка завершена. Модуль " ("string"), w217) -> (w225:string)
      n140 = call "Send Write to Module.vi"("Data"=w206, "Module"=enum16{"LAI", "LDO", "Control"}."LDO", "Message Enqueuer"=w207) -> ()  [unwired: 7 in, 2 out]
      n141 = property class="Str"(reference=w216, "Value"=w225) -> (error out=w214:errorcluster)  [unwired: 1 in, 1 out]
      n142 = call <vilib>:"Send Normal Stop.vi"("error in (no error)"=w214, "Message Enqueuer"=w213) -> ("error out"=w212:errorcluster)  [unwired: 9 in]
      n143 = call "Send Get Alg Result.vi"("Alg result"=w210, "Message Enqueuer"=w209) -> ()  [unwired: 8 in, 2 out]
      n144 = call <vilib>:"Clear Errors.vi"("error in (no error)"=w212) -> ()  [unwired: 5 in, 2 out]
    }
  }
